vi "PH_Img_BaseClass.contents.vi"   [LabVIEW 2014, in "PH_Img_BaseClass.lvlib"]
doc: "This class is forseen to xxx\n\nThis class is part of the PHELIX xxx layer."
uses:
  PH_Img_BaseClass.lvlib
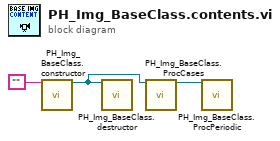
[diagram p0: block diagram]
diagram:
  n1 = call "PH_Img_BaseClass.constructor.vi"("name"="") -> ("i ref out"=w1:refnum<vi>)  [unwired: 16 in, 2 out]
  n2 = call "PH_Img_BaseClass.destructor.vi"("i ref in"=w1) -> ()  [unwired: 18 in, 1 out]
  n3 = call "PH_Img_BaseClass.ProcCases.vi"("i ref in"=w1) -> ("i ref out"=w2:refnum<vi>)  [unwired: 16 in, 2 out]
  n4 = call "PH_Img_BaseClass.ProcPeriodic.vi"("i ref in"=w2) -> ()  [unwired: 14 in, 5 out]
